vi "write Could (subVi).vi"(8 "Array":cluster{"X (m)":sgl, "Y (m)":sgl}[](array[cluster]), 10 "Experiment":path, 11 "Experiment Name":string) -> ()   [LabVIEW 2014]
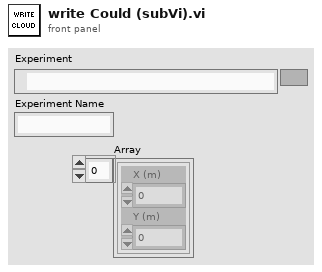
[diagram p1: front panel]
types:
  T1 = enum16{"open", "replace", "create", "open or create", "replace or create", "replace or create with confirmation"}
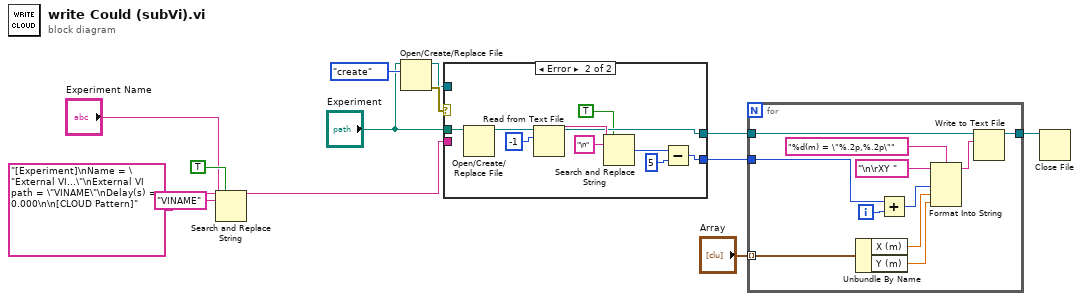
[diagram p0: block diagram]
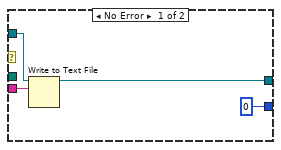
[diagram p2: hidden frame]
diagram:
  n1 = Search and Replace String(replace all?=TRUE ("replace all? (F)"), input string="[Experiment]\nName = \"External VI...\"\nExternal VI path = \"VINAME\"\nDelay(s) = 0.000\n\n[CLOUD Pattern]", search string="VINAME", replace string="Experiment Name") -> (result string=w4:string)  [unwired: 4 in, 3 out]
  n2 = Open/Create/Replace File(file path (use dialog)="Experiment", operation (0:open)=T1."create") -> (refnum out=w11:refnum<file>, error out=w12:errorcluster)  [unwired: 4 in, 1 out]
  n3 = case shown="Error" w12 {
    tunnel: w11 -> [w17 _]
    tunnel: "Experiment" -> [_ w21]
    tunnel: w4 -> [w16 _]
    tunnel: [0 w24] -> w8
    tunnel: [w14 w20] -> w7
    frame No Error {
      n4 = Write to Text File(file (use dialog)=w17, text=w16) -> (refnum out=w14:refnum<file>)  [unwired: 2 in, 2 out]
    }
    frame Error {
      n5 = Open/Create/Replace File(file path (use dialog)=w21) -> (refnum out=w27:refnum<file>)  [unwired: 5 in, 2 out]
      n6 = Read from Text File(file (use dialog)=w27, count=-1) -> (refnum out=w20:refnum<file>, text=w25:string)  [unwired: 2 in, 2 out]
      n7 = Search and Replace String(replace all?=TRUE ("replace all? (F)"), input string=w25, search string="\n") -> (number of replacements=w23:i32)  [unwired: 5 in, 3 out]
      n8 = Subtract(x=w23, y=5) -> (x-y=w24:i32)
    }
  }
  n9 = for {
    tunnel: "Array" -> [w30] mode=indexing
    tunnel: w8 -> [w38]
    tunnel: w7 -> [w36]
    tunnel: [w31] -> w6
    i -> [w37]
    n10 = Unbundle By Name(w30) -> ("X (m)"=w29:sgl, "Y (m)"=w28:sgl)
    n11 = Add(x=w38, y=w37) -> (x+y=w33:i32)
    n12 = Format Into String(format string="%d(m) = \"%.2p,%.2p\"", initial string="\n\rXY ", w33, w29, w28) -> (resulting string=w32:string)  [unwired: 1 in, 1 out]
    n13 = Write to Text File(file (use dialog)=w36, text=w32) -> (refnum out=w31:refnum<file>)  [unwired: 2 in, 2 out]
  }
  n14 = Close File(refnum=w6) -> ()  [unwired: 1 in, 2 out]
